vi "CloseConfigFile.vi"(8 "error in (no error)":errorcluster, 10 "refnum":T1, 11 "GRMActor in":refnum<class "GeneralRMActor.lvclass">) -> (0 "error out":errorcluster, 3 "GRMActor out":refnum<class "GeneralRMActor.lvclass">)   [LabVIEW 2020, in "GeneralRMActor.lvlib" / "GeneralRMActor.lvclass"]
uses:
  GeneralRMActor.lvclass
  <vilib>/Utility/config.llb/Config Data RefNum.ctl
  <vilib>/Utility/config.llb/NI_LVConfig.lvlib
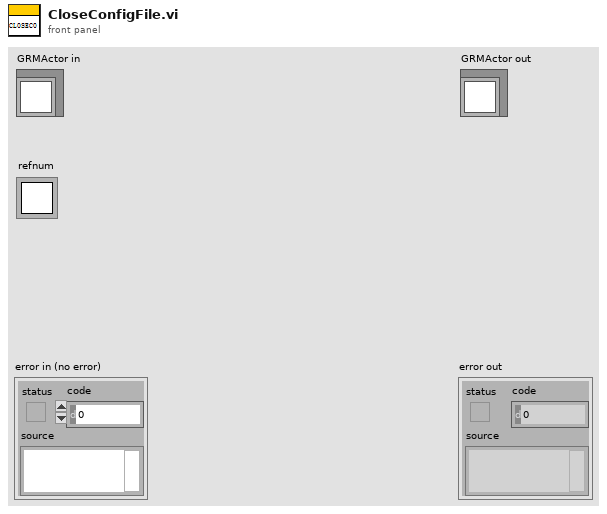
[diagram p1: front panel]
types:
  T1 = typedef "NI_LVConfig.lvlib/Config Data RefNum.ctl" = refnum<k1>
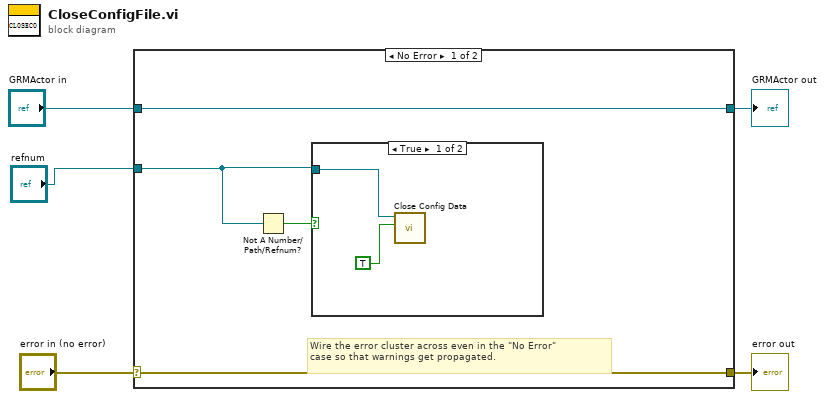
[diagram p0: block diagram]
diagram:
  n1 = case shown="No Error" "error in (no error)" {
    selector: "error in (no error)" -> [w8 w13]
    tunnel: [w8 w13] -> w4
    tunnel: [w9 w12] -> w2
    tunnel: "GRMActor in" -> [w9 w12]
    tunnel: "refnum" -> [w6 _]
    frame No Error {
      # "Wire the error cluster across even in the \"No Error\"\ncase so that warnings get propagated."
      n2 = Not A Number/Path/Refnum?(number/path/refnum=w6) -> (NaN/Path/Refnum?=w7:bool)
      n3 = case shown="True" w7 {
        tunnel: w6 -> [w10 _]
        frame True {
          n4 = call <vilib>:"Close Config Data.vi"("write file if changed (T)"=TRUE, "refnum"=w10) -> ()  [unwired: 8 in, 2 out]
        }
        frame False {
        }
      }
    }
    frame Error {
    }
  }
  "error out" <- w4
  "GRMActor out" <- w2
